vi "Plot init scales GUI.vi"(4 "Right axis":refnum<vi>, 6 "Left axis":refnum<vi>, 8 "error in (no error)":errorcluster, 10 "X-axis":refnum<vi>, 11 "Plot config":T2={"plots"=[], "X-axis"={"Name Label.Text"="", "Style"=0, "Tick Colors:Minor Tick Color"=0, "Tick Colors:Tick Color"=0, "Marker Colors:Text Color"=0, "Grid Colors:Major Color"=0, "Grid Colors:Minor Color"=0, "Mapping Mode"=0, "Flipped"=FALSE, "Name Label.Visible"=FALSE, "Name Label.Text Colors:Text Color"=0, "Scale Fit"=0, "Range:Maximum"=0.0, "Range:Minimum"=0.0, "Offset and Multiplier:Multiplier"=0.0, "Offset and Multiplier:Offset"=0.0, "Name Label.Font:Size"=0, "Marker.Font:Size"=0, "Uniform Marker Spacing?"=TRUE, "Format String"=""}, "Y-axes"=[], "General"={"Title"="", "Time to Plot"=1800.0, "Title.Visible"=FALSE, "Sidebar.Visible"=FALSE, "Plot Area:Colors:BG Color"=0, "X Scale.Plot Name"="", "X Scale.Use Plot Name"=FALSE}} {"General"."Time to Plot" format="%<%M:%S>t"}) -> (0 "error out":errorcluster, 2 "axis SubRefs":T1[](array[typedef]), 3 "Axis references":refnum<vi>[](array[refnum]))   [LabVIEW 2021, in "RocketPlot.lvlib"]
uses:
  RocketPlot.lvlib
  TypeDefs/plot load data V2.ctl
  TypeDefs/plot properties V2.ctl
  TypeDefs/plot attributes V2.ctl
  TypeDefs/Plot scale axis properties.ctl
  TypeDefs/Plot general properties.ctl
  TypeDefs/Plot axis GUI.ctl
  tick style/plot tick style picture ring.ctl
  lock/plot lock button.ctl
  horiz grid/plot horizontal grid pic ring.ctl
  vert grid/plot vertical grid pic ring.ctl
  TypeDefs/Plot axis gui refs.ctl
panel:
  # "Scaling Factors"
  # "Font Sizes"
  # "Scaling Factors"
  # "Font Sizes"
  # "Scaling Factors"
  # "Font Sizes"
  # "Scaling Factors"
  # "Font Sizes"
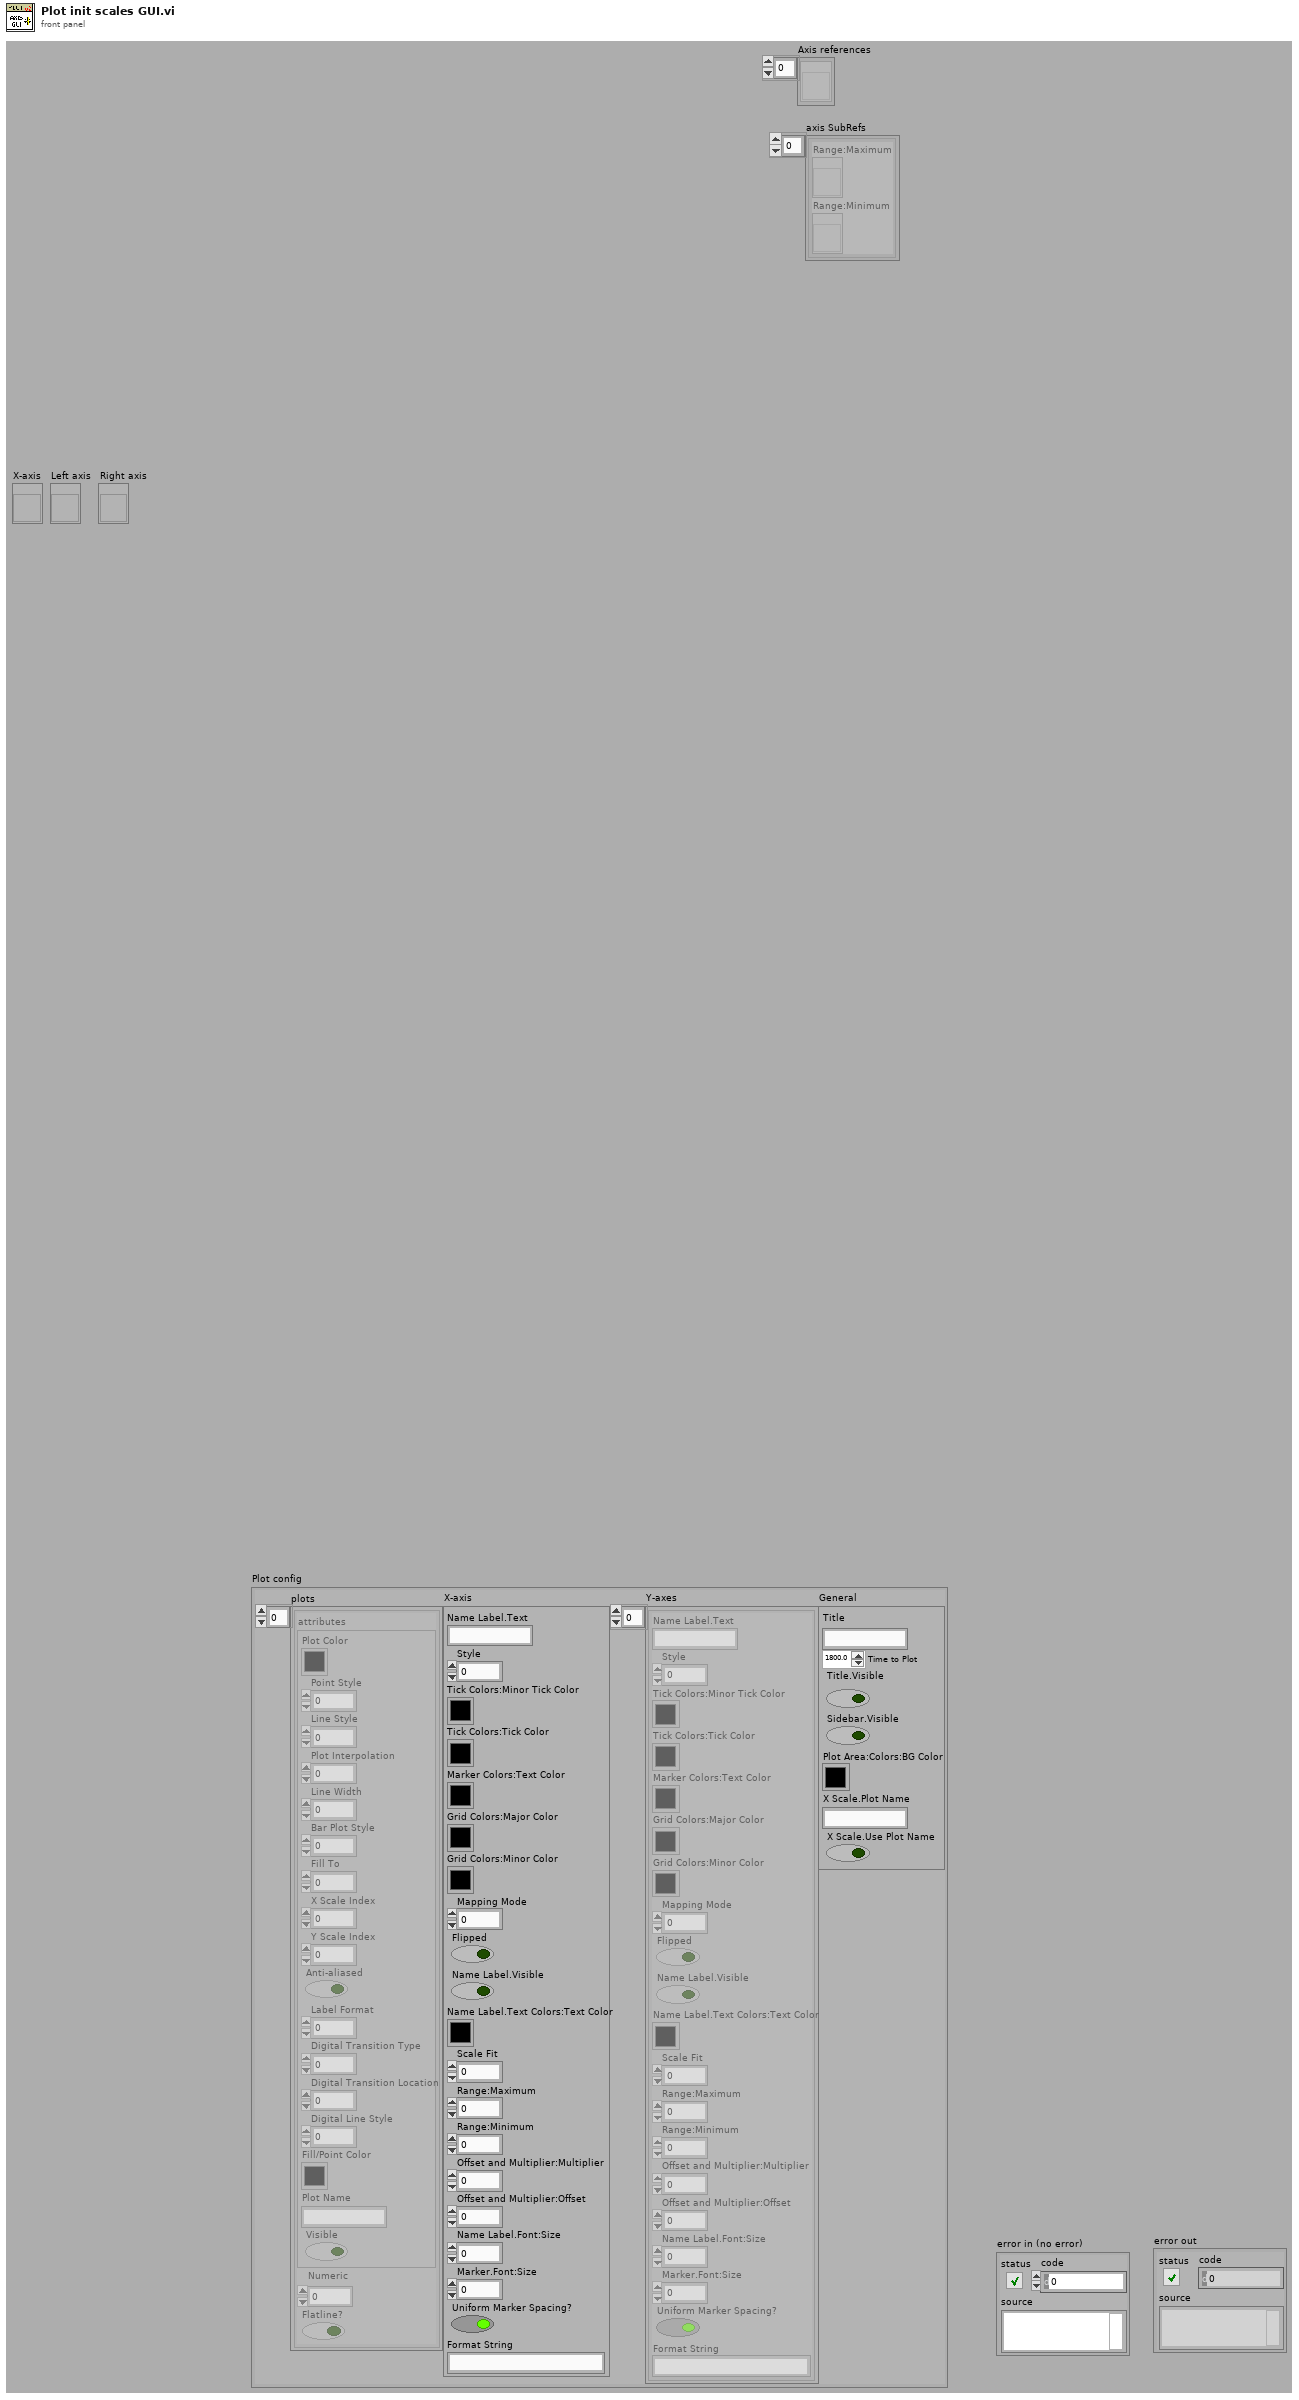
[diagram p1: front panel]
types:
  T1 = typedef "RocketPlot.lvlib/Plot axis gui refs.ctl" = cluster{"Range:Maximum":refnum<vi>, "Range:Minimum":refnum<vi>}
  T2 = typedef "RocketPlot.lvlib/plot load data V2.ctl" = cluster{"plots":T3[], "X-axis":T5, "Y-axes":T5[], "General":T6}
  T3 = typedef "RocketPlot.lvlib/plot properties V2.ctl" = cluster{"attributes":T4, "Numeric":dbl, "Flatline?":bool}
  T4 = typedef "RocketPlot.lvlib/plot attributes V2.ctl" = cluster{"Plot Color":u32, "Point Style":u8, "Line Style":u8, "Plot Interpolation":u8, "Line Width":u8, "Bar Plot Style":u8, "Fill To":i16, "X Scale Index":u32, "Y Scale Index":u32, "Anti-aliased":bool, "Label Format":u8, "Digital Transition Type":u8, "Digital Transition Location":u8, "Digital Line Style":u8, "Fill/Point Color":u32, "Plot Name":string, "Visible":bool}
  T5 = typedef "RocketPlot.lvlib/Plot scale axis properties.ctl" = cluster{"Name Label.Text":string, "Style":u8, "Tick Colors:Minor Tick Color":u32, "Tick Colors:Tick Color":u32, "Marker Colors:Text Color":u32, "Grid Colors:Major Color":u32, "Grid Colors:Minor Color":u32, "Mapping Mode":u8, "Flipped":bool, "Name Label.Visible":bool, "Name Label.Text Colors:Text Color":u32, "Scale Fit":u8, "Range:Maximum":dbl, "Range:Minimum":dbl, "Offset and Multiplier:Multiplier":dbl, "Offset and Multiplier:Offset":dbl, "Name Label.Font:Size":u32, "Marker.Font:Size":u32, "Uniform Marker Spacing?":bool, "Format String":string}
  T6 = typedef "RocketPlot.lvlib/Plot general properties.ctl" = cluster{"Title":string, "Time to Plot":dbl, "Title.Visible":bool, "Sidebar.Visible":bool, "Plot Area:Colors:BG Color":u32, "X Scale.Plot Name":string, "X Scale.Use Plot Name":bool}
  T7 = enum8{"Enabled", "Disabled", "Disabled and Grayed Out"}
  T8 = typedef "RocketPlot.lvlib/Plot axis GUI.ctl" = cluster{"Tick Colors:Tick Color":u32, "Tick Colors:Minor Tick Color":u32, "Name Label.Text":string, "Marker Colors:Text Color":u32, "Name Label.Font:Size":string, "Marker.Font:Size":string, "Flipped":bool, "Tick Style":T9, "Grid Colors:Major Color":u32, "Grid Colors:Minor Color":u32, "Mapping Mode":bool, "Autoscale?":T10, "Range:Minimum":dbl, "Range:Maximum":dbl, "Offset and Multiplier:Multiplier":dbl, "Offset and Multiplier:Offset":dbl, "Horiz.Grid Style":T11, "Name Label.Text Colors:Text Color":u32, "Vert.Grid Style":T12, "Name Label.Visible":bool, "Uniform Marker Spacing?":bool, "Format String":string}
  T9 = typedef "RocketPlot.lvlib/plot tick style picture ring.ctl" = u16
  T10 = typedef "RocketPlot.lvlib/plot lock button.ctl" = bool
  T11 = typedef "RocketPlot.lvlib/plot horizontal grid pic ring.ctl" = u16
  T12 = typedef "RocketPlot.lvlib/plot vertical grid pic ring.ctl" = u16
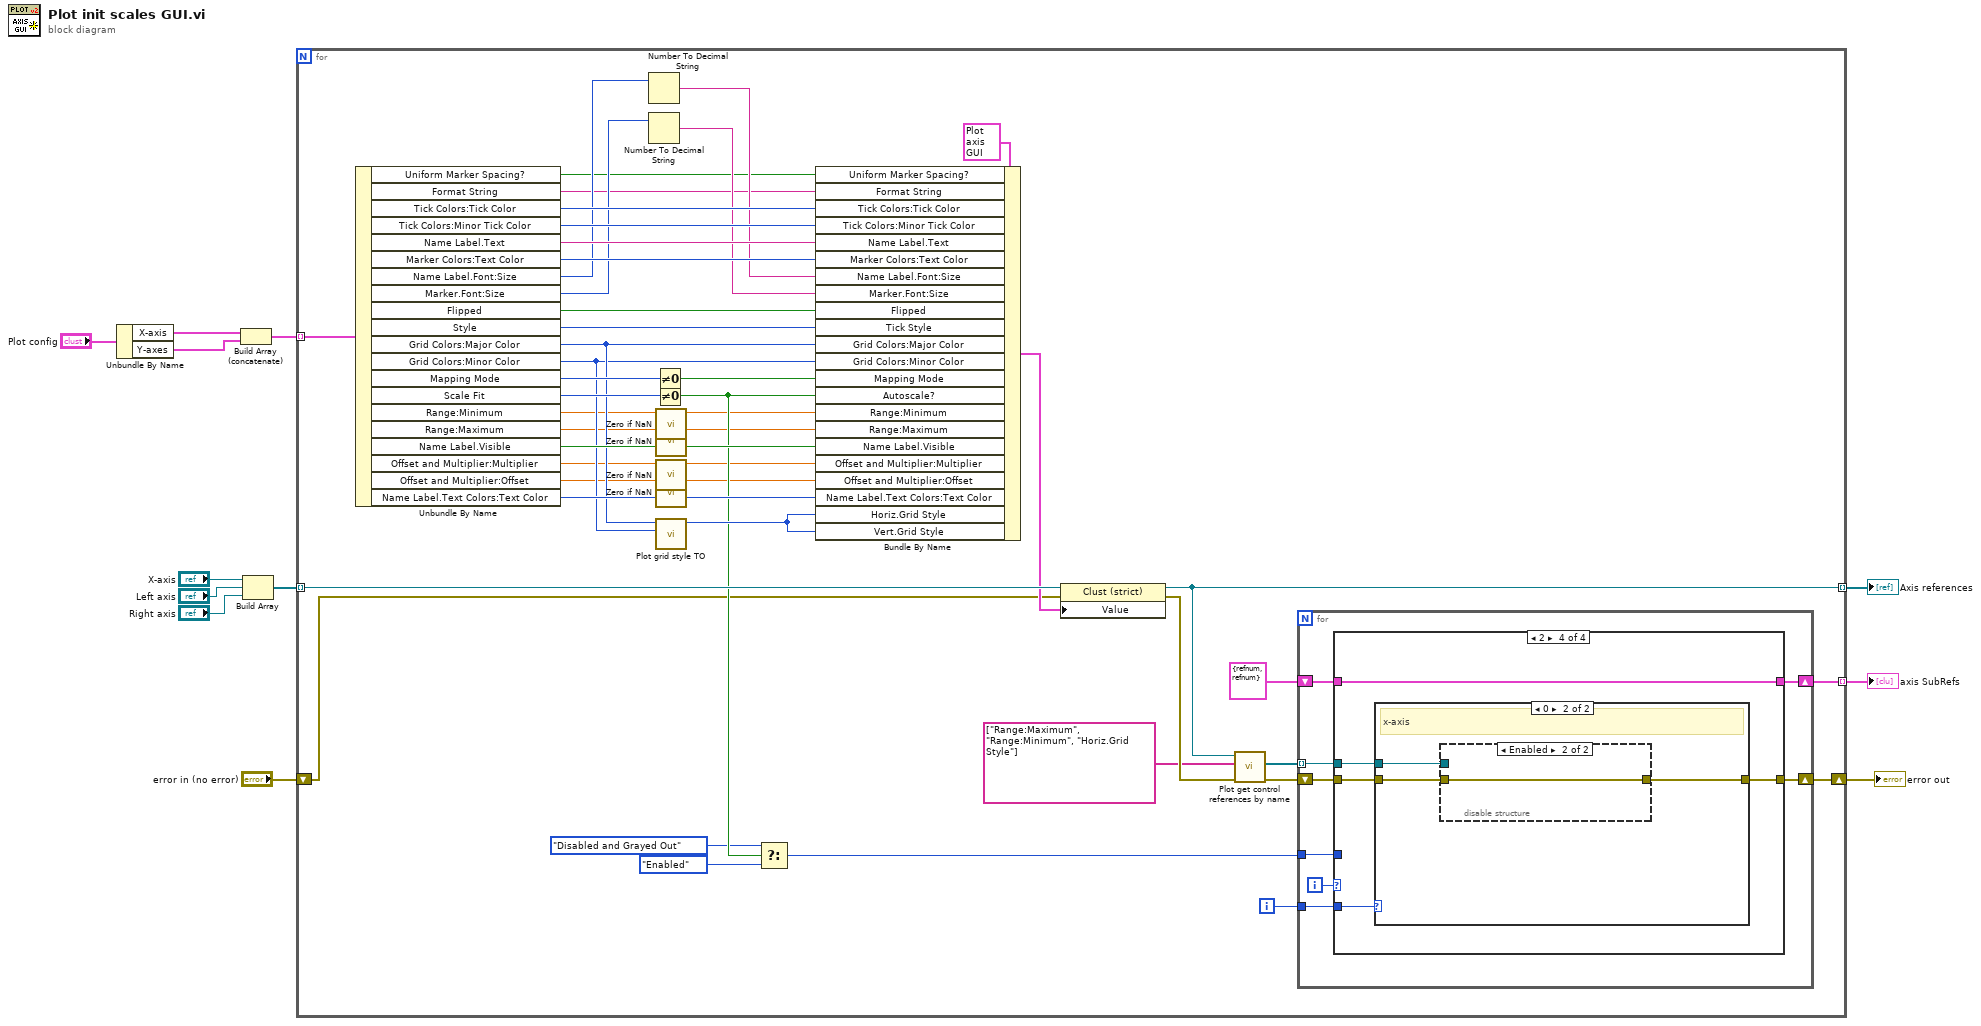
[diagram p0: block diagram]
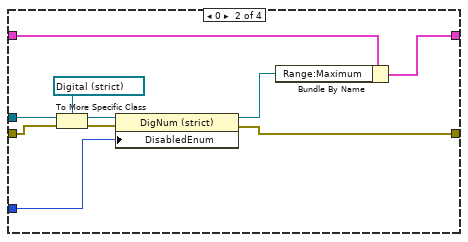
[diagram p3: hidden frame]
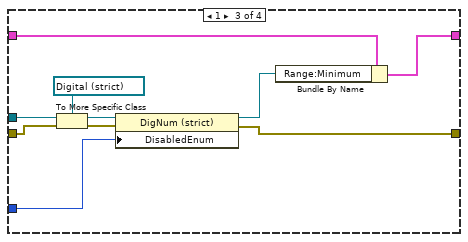
[diagram p4: hidden frame]
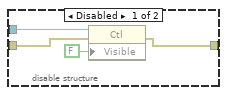
[diagram p6: hidden frame]
diagram:
  n1 = Unbundle By Name("Plot config") -> ("X-axis"=w11:T5, "Y-axes"=w10:T5[])
  n2 = Build Array (concatenate)(w11, w10) -> (w9:T5[])
  n3 = Build Array("X-axis", "Left axis", "Right axis") -> (w5:refnum<vi>[])
  n4 = for {
    tunnel: w9 -> [w39] mode=indexing
    tunnel: w5 -> [w38] mode=indexing
    tunnel: [w35] -> w4 mode=indexing
    shift-right: [w25] -> w1
    shift-left: "error in (no error)" -> [w24]
    tunnel: [w23] -> w2 mode=indexing
    i -> [w27]
    n5 = Unbundle By Name(w39) -> ("Uniform Marker Spacing?"=w13:bool, "Format String"=w14:string, "Tick Colors:Tick Color"=w57:u32, "Tick Colors:Minor Tick Color"=w56:u32, "Name Label.Text"=w55:string, "Marker Colors:Text Color"=w54:u32, "Name Label.Font:Size"=w53:u32, "Marker.Font:Size"=w51:u32, "Flipped"=w49:bool, "Style"=w48:u8, "Grid Colors:Major Color"=w42:u32, "Grid Colors:Minor Color"=w41:u32, "Mapping Mode"=w47:u8, "Scale Fit"=w45:u8, "Range:Minimum"=w22:dbl, "Range:Maximum"=w21:dbl, "Name Label.Visible"=w44:bool, "Offset and Multiplier:Multiplier"=w20:dbl, "Offset and Multiplier:Offset"=w19:dbl, "Name Label.Text Colors:Text Color"=w43:u32)
    n6 = Number To Decimal String(number=w53) -> (decimal integer string=w52:string)  [unwired: 1 in]
    n7 = Number To Decimal String(number=w51) -> (decimal integer string=w50:string)  [unwired: 1 in]
    n8 = Not Equal To 0?(x=w47) -> (x != 0?=w46:bool)
    n9 = Not Equal To 0?(x=w45) -> (x != 0?=w31:bool)
    n10 = call "Zero if NaN.vi"("Numeric"=w22) -> ("Numeric"=w18:dbl)  [unwired: 10 in]
    n11 = call "Zero if NaN.vi"("Numeric"=w21) -> ("Numeric"=w17:dbl)  [unwired: 10 in]
    n12 = call "Zero if NaN.vi"("Numeric"=w20) -> ("Numeric"=w16:dbl)  [unwired: 10 in]
    n13 = call "Zero if NaN.vi"("Numeric"=w19) -> ("Numeric"=w15:dbl)  [unwired: 10 in]
    n14 = call "Plot grid style TO.vi"("Grid Colors:Minor Color"=w41, "Grid Colors:Major Color"=w42) -> ("Grid Style"=w40:T11)  [unwired: 9 in]
    n15 = Select(t=T7."Disabled and Grayed Out" ("Disabled"), s=w31, f=T7."Enabled" ("Disabled")) -> (s? t:f=w28:T7)
    n16 = Bundle By Name(cluster=T8 {"Tick Colors:Tick Color"=4294967295, "Tick Colors:Minor Tick Color"=4294967295, "Name Label.Text"="", "Marker Colors:Text Color"=16777225, "Name Label.Font:Size"="", "Marker.Font:Size"="", "Flipped"=FALSE, "Tick Style"=0, "Grid Colors:Major Color"=0, "Grid Colors:Minor Color"=0, "Mapping Mode"=FALSE, "Autoscale?"=FALSE, "Range:Minimum"=0.0, "Range:Maximum"=0.0, "Offset and Multiplier:Multiplier"=0.0, "Offset and Multiplier:Offset"=0.0, "Horiz.Grid Style"=0, "Name Label.Text Colors:Text Color"=0, "Vert.Grid Style"=0, "Name Label.Visible"=FALSE, "Uniform Marker Spacing?"=FALSE, "Format String"=""} ("X-axis"), "Uniform Marker Spacing?"=w13, "Format String"=w14, "Tick Colors:Tick Color"=w57, "Tick Colors:Minor Tick Color"=w56, "Name Label.Text"=w55, "Marker Colors:Text Color"=w54, "Name Label.Font:Size"=w52, "Marker.Font:Size"=w50, "Flipped"=w49, "Tick Style"=w48, "Grid Colors:Major Color"=w42, "Grid Colors:Minor Color"=w41, "Mapping Mode"=w46, "Autoscale?"=w31, "Range:Minimum"=w18, "Range:Maximum"=w17, "Name Label.Visible"=w44, "Offset and Multiplier:Multiplier"=w16, "Offset and Multiplier:Offset"=w15, "Name Label.Text Colors:Text Color"=w43, "Horiz.Grid Style"=w40, "Vert.Grid Style"=w40) -> (w37:T8)
    n17 = property class="Clust (strict)"(reference=w38, error in=w24, "Value"=w37) -> (reference out=w35:refnum<vi>, error out=w36:errorcluster)
    n18 = call "Plot get control references by name.vi"("error in (no error)"=w36, "Control label names"=string[] ["Range:Maximum", "Range:Minimum", "Horiz.Grid Style"], "Cluster reference"=w35) -> ("error out"=w26:errorcluster, "Controls[]"=w33:refnum<vi>[])  [unwired: 7 in]
    n19 = for {
      tunnel: w33 -> [w66] mode=indexing
      shift-right: [w64] -> w23
      shift-left: T1 {"Range:Maximum"=refnum, "Range:Minimum"=refnum} -> [w65]
      tunnel: w28 -> [w63]
      tunnel: w27 -> [w61]
      shift-right: [w59] -> w25
      shift-left: w26 -> [w60]
      i -> [w62]
      n20 = case shown="2" w62 {
        tunnel: w66 -> [_ w78 w88 w91]
        tunnel: w65 -> [w67 w76 w86 w93]
        tunnel: [w67 w75 w85 w93] -> w64
        tunnel: w63 -> [_ w72 w82 _]
        tunnel: w61 -> [_ _ _ w92]
        tunnel: w60 -> [w68 w71 w81 w90]
        tunnel: [w68 w69 w79 w89] -> w59
        frame Default {
        }
        frame 0 {
          n21 = To More Specific Class(target class=refnum<vi> refnum ("Range:Maximum"), reference=w78, error in=w71) -> (specific class reference=w74:refnum<vi>, error out=w70:errorcluster)
          n22 = property class="DigNum (strict)"(reference=w74, error in=w70, "DisabledEnum"=w72) -> (reference out=w73:refnum<vi>, error out=w69:errorcluster)
          n23 = Bundle By Name(cluster=w76, "Range:Maximum"=w73) -> (w75:T1)
        }
        frame 1 {
          n24 = To More Specific Class(target class=refnum<vi> refnum ("Range:Maximum"), reference=w88, error in=w81) -> (specific class reference=w84:refnum<vi>, error out=w80:errorcluster)
          n25 = property class="DigNum (strict)"(reference=w84, error in=w80, "DisabledEnum"=w82) -> (reference out=w83:refnum<vi>, error out=w79:errorcluster)
          n26 = Bundle By Name(cluster=w86, "Range:Minimum"=w83) -> (w85:T1)
        }
        frame 2 {
          n27 = case shown="0" w92 {
            tunnel: w91 -> [_ w97]
            tunnel: w90 -> [w94 w96]
            tunnel: [w94 w95] -> w89
            frame Default {
              # "y-axes"
            }
            frame 0 {
              # "x-axis"
              n28 = disable-structure shown="Enabled" {
                disable-tunnel: w97 -> [w101 _]
                disable-tunnel: w96 -> [w99 w102]
                disable-tunnel: [w98 w102] -> w95
                frame Disabled {
                  n29 = property class="Ctl"(reference=w101, error in=w99, "Visible"=FALSE) -> (error out=w98:errorcluster)  [unwired: 1 out]
                }
                frame Enabled {
                }
              }
            }
          }
        }
      }
    }
  }
  "error out" <- w1
  "Axis references" <- w4
  "axis SubRefs" <- w2
